vi "Set Trigger Input High or Low.vi"(8 "error in":errorcluster, 9 "Level":bool, 10 "Line":tag="Dev1/port0/line0") -> (0 "error out":errorcluster)   [LabVIEW 2016, in "2P Trigger.lvlib"]
doc: "This example demonstrates how to generate a finite amount of digital data based off of a sample clock.\n\nSome hardware (e.g. M Series DAQ) must use an external sample clock for digital tasks. To view a complete list of available sample clock sources, consult the Device Routes table in Measurement and Automation Explorer.\n\nFor instructions on how to connect your signals to the DAQ device, refer to your device documentation."
uses:
  2P Trigger.lvlib
  <vilib>/DAQmx/write.llb/DAQmx Write (Digital Bool 1Line 1Point).vi
  <vilib>/DAQmx/create/channels.llb/DAQmx Create Channel (DO-Digital Output).vi
  <vilib>/DAQmx/configure/trigger.llb/DAQmx Start Trigger (Digital Edge).vi
  <vilib>/DAQmx/miscellaneous.llb/DAQmx Fill In Error Info.vi
panel:
  in  "Trigger Type":enum32{"No Trigger", "Digital Start"}(tab)
  in  "Edge":i32(ring)=10280 items=["Rising"=10280, "Falling"=10171]
  in  "Digital Trigger Source":tag="PFI1"
  # "Channel Settings"
  # "Data to Write"
  # "High\n\nLow"
  # "Timing and Buffer Settings"
  # "Trigger Settings"
  # "To configure and use a start trigger you must have the necessary tab selected above.  Not all hardware supports triggering--refer to your device documentation for more info."
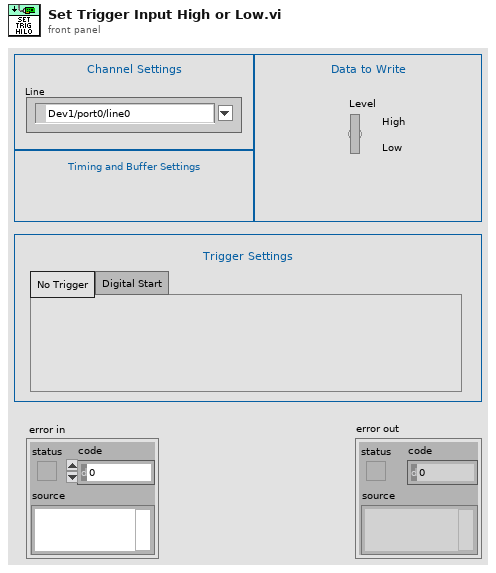
[diagram p1: front panel]
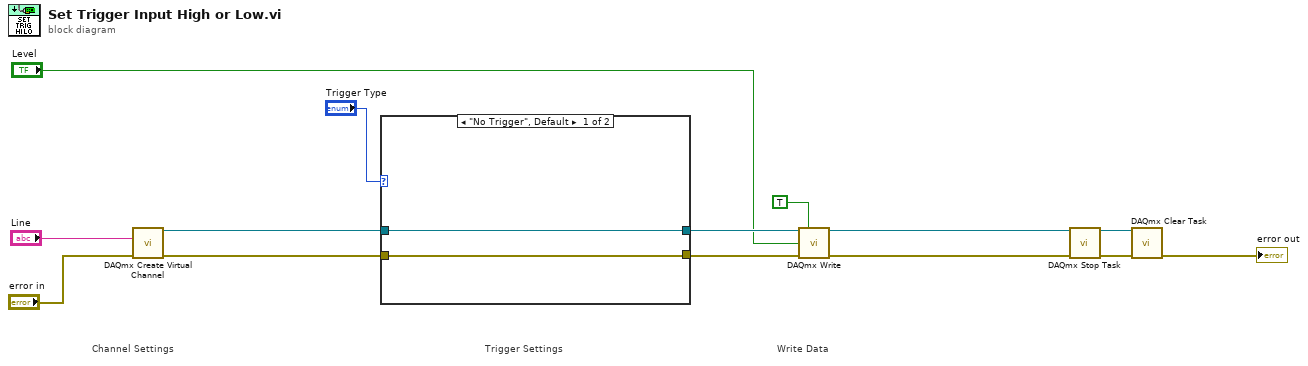
[diagram p0: block diagram]
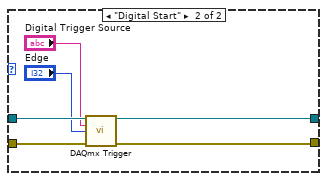
[diagram p2: hidden frame]
diagram:
  # "Trigger Settings"
  # "Write Data"
  # "Channel Settings"
  n1 = call-poly <vilib>:"DAQmx Create Virtual Channel.vi"("lines"="Line", "error in"="error in") -> ("task out"=w7:refnum<k21>, "error out"=w6:errorcluster)  [unwired: 12 in]
  n2 = case shown="\"No Trigger\", Default" "Trigger Type" {
    tunnel: w7 -> [w16 w22]
    tunnel: w6 -> [w15 w21]
    tunnel: [w16 w20] -> w11
    tunnel: [w15 w19] -> w10
    frame "No Trigger", Default {
    }
    frame "Digital Start" {
      n3 = call-poly <vilib>:"DAQmx Trigger.vi"("task/channels in"=w22, "source"="Digital Trigger Source", "edge"="Edge", "error in"=w21) -> ("task out"=w20:refnum<k21>, "error out"=w19:errorcluster)  [unwired: 10 in]
    }
  }
  n4 = call-poly <vilib>:"DAQmx Write.vi"("task/channels in"=w11, "auto start"=TRUE, "data"="Level", "error in"=w10) -> ("task out"=w4:refnum<k21>, "error out"=w3:errorcluster)  [unwired: 9 in, 1 out]
  n5 = call <vilib>:"DAQmx Stop Task.vi"("task/channels in"=w4, "error in"=w3) -> ("task out"=w9:refnum<k21>, "error out"=w8:errorcluster)  [unwired: 12 in]
  n6 = call <vilib>:"DAQmx Clear Task.vi"("task in"=w9, "error in"=w8) -> ("error out"=→"error out":errorcluster)  [unwired: 13 in]
